vi "Write Graph Reference.vi"(8 "error in (no error)":errorcluster, 10 "Graph":refnum<vi>, 11 "PowerSupply in":refnum<class "PowerSupply.lvclass">) -> (0 "error out":errorcluster, 3 "PowerSupply out":refnum<class "PowerSupply.lvclass">)   [LabVIEW 2019]
uses:
  Library/PowerSupply.lvclass
  Library/PowerSupply.lvclass/PowerSupply.ctl
  C:/Users/Public/Documents/Development/builds/Instruments/Instruments.lvlibp/Library/Instruments.lvclass
  C:/Users/Public/Documents/Development/builds/Tools/Config.lvlibp/Config.lvclass
  C:/Users/Public/Documents/Development/builds/Engine/Engine.lvlibp/Project/Engine.lvclass
  C:/Users/Public/Documents/Development/builds/Engine/Panel Manager.lvlibp/Panel Actor/Panel Actor.lvclass
  C:/Users/Public/Documents/Development/builds/Engine/Monitored Actor.lvlibp/Monitored Actor/Monitored Actor/Monitored Actor.lvclass
  C:/Users/Public/Documents/Development/builds/Engine/Actor Framework.lvlibp/1abvi3w/vi.lib/ActorFramework/Actor/Actor.lvclass
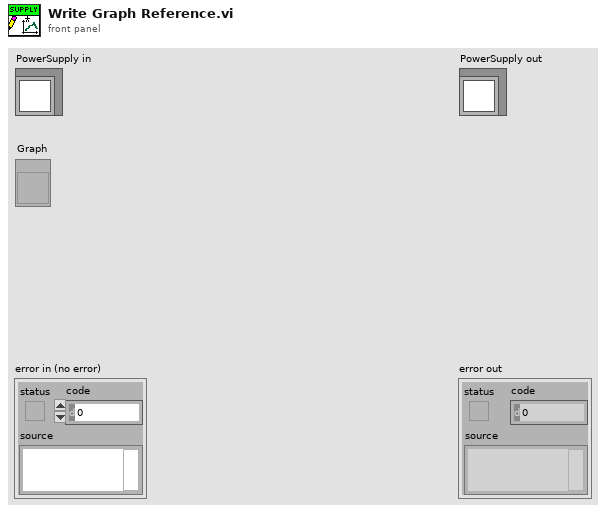
[diagram p1: front panel]
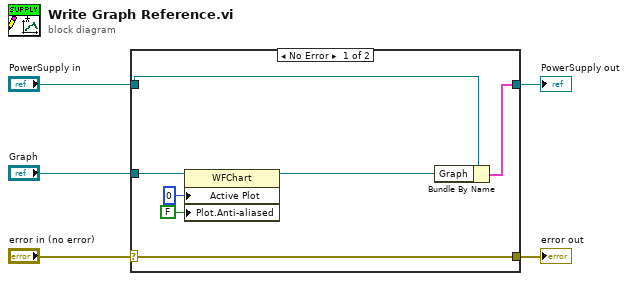
[diagram p0: block diagram]
diagram:
  n1 = case shown="No Error" "error in (no error)" {
    selector: "error in (no error)" -> [w12 w13]
    tunnel: [w12 w13] -> w4
    tunnel: [w10 w14] -> w2
    tunnel: "PowerSupply in" -> [w11 w14]
    tunnel: "Graph" -> [w9 _]
    frame No Error {
      n2 = property class="WFChart"(reference=w9, "Active Plot"=u32 0, "Plot.Anti-aliased"=FALSE) -> (reference out=w8:refnum<vi>)  [unwired: 1 in, 1 out]
      n3 = Bundle By Name(cluster=w11, "Graph"=w8) -> (w10:cluster{})
    }
    frame Error {
    }
  }
  "error out" <- w4
  "PowerSupply out" <- w2
